vi "Read Measurement.vi"(8 "error in (no error)":errorcluster, 10 "Display (0: Primary)":i32(ring) items=["Primary", "Secondary", "Both"], 11 "VISA resource name":refnum<visa-resource-name>) -> (0 "error out":errorcluster, 1 "Secondary Measurement":dbl, 2 "Primary Measurement":dbl, 3 "VISA resource name out":refnum<visa-resource-name>)   [LabVIEW 2021, in "GWInstek  GDM8351.lvlib"]
doc: "Read the Primary or Secondary display from the instument."
uses:
  <instrlib>/GWInstek  GDM8351/GWInstek  GDM8351.lvlib
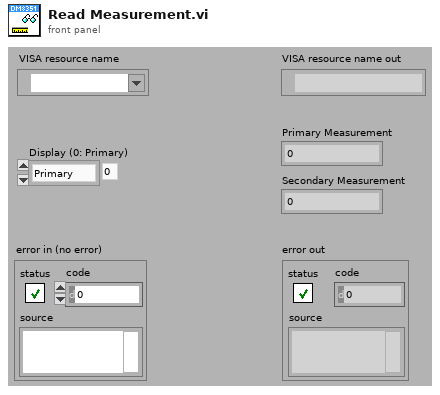
[diagram p1: front panel]
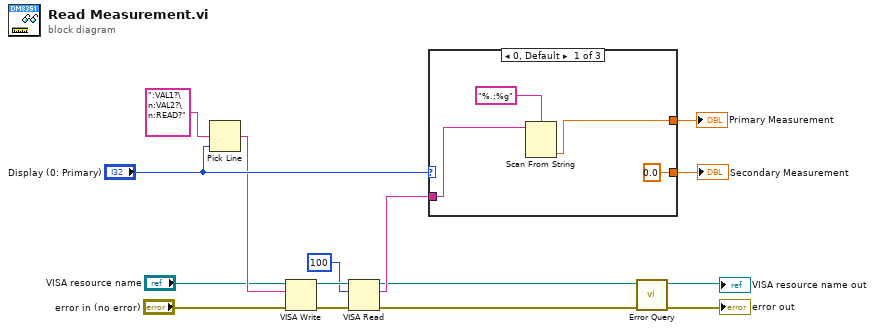
[diagram p0: block diagram]
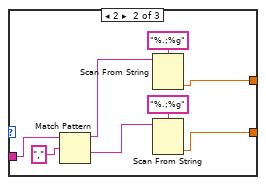
[diagram p2: hidden frame]
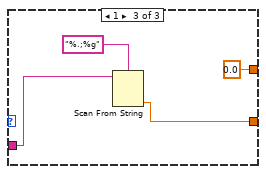
[diagram p3: hidden frame]
diagram:
  n1 = Pick Line(multi-line string=":VAL1?\n:VAL2?\n:READ?", line index="Display (0: Primary)") -> (output string=w13:string)  [unwired: 1 in]
  n2 = VISA Write(VISA resource name="VISA resource name", write buffer=w13, error in (no error)="error in (no error)") -> (VISA resource name out=w10:refnum<visa-resource-name>, error out=w9:errorcluster)  [unwired: 1 out]
  n3 = VISA Read(VISA resource name=w10, byte count=u32 100, error in (no error)=w9) -> (VISA resource name out=w2:refnum<visa-resource-name>, read buffer=w7:string, error out=w1:errorcluster)  [unwired: 1 out]
  n4 = case shown="0, Default" "Display (0: Primary)" {
    tunnel: w7 -> [w19 w27 w31]
    tunnel: [w17 w22 0.0] -> w6
    tunnel: [0.0 w21 w29] -> w5
    frame 0, Default {
      n5 = Scan From String(format string="%.;%g", input string=w19) -> (output 1=w17:dbl)  [unwired: 3 in, 3 out]
    }
    frame 2 {
      n6 = Match Pattern(string=w27, regular expression=",") -> (before substring=w25:string, after substring=w24:string)  [unwired: 1 in, 2 out]
      n7 = Scan From String(format string="%.;%g", input string=w25) -> (output 1=w22:dbl)  [unwired: 3 in, 3 out]
      n8 = Scan From String(format string="%.;%g", input string=w24) -> (output 1=w21:dbl)  [unwired: 3 in, 3 out]
    }
    frame 1 {
      n9 = Scan From String(format string="%.;%g", input string=w31) -> (output 1=w29:dbl)  [unwired: 3 in, 3 out]
    }
  }
  "Primary Measurement" <- w6
  "Secondary Measurement" <- w5
  n10 = call <instrlib>:"Error Query.vi"("error in (no error)"=w1, "VISA resource name"=w2) -> ("error out"=→"error out":errorcluster, "VISA resource name out"=→"VISA resource name out":refnum<visa-resource-name>)  [unwired: 6 in, 2 out]
